vi "Main.vi"(0 "Start":bool, 1 "Temperature_Limit":T2={"Temperature_High_limit"=50.0, "Temperature_Low_Limit"=30.0} {"Temperature_Low_Limit" min=30.0 max=50.0 step=1.0; "Temperature_High_limit" min=30.0 max=50.0 step=1.0}, 2 "Current_Limit":T1={"Current_High_Limit"=120.0, "Current_Low_Limit"=100.0} {"Current_Low_Limit" min=100.0 max=120.0 step=1.0; "Current_High_Limit" min=100.0 max=120.0 step=1.0}, 5 "Stop":bool, 7 "Exit":bool, 9 "Log Rate":dbl, 11 "Error in":errorcluster) -> (4 "Temperature":i32, 6 "Current":i32, 8 "Waveform Graph":dbl[][](graph), 15 "Error out":errorcluster)   [LabVIEW 2020]
doc: "This system is used to get the current and temperature data which is generated and check if the generated data is in the specific range and generate error and the data is logged in the graph and the user can customize the the time on which the graph to be plotted"
uses:
  Controls/Temperature limit.ctl
  Controls/Current limit.ctl
  Typedefs/Data cluster.ctl
  Typedefs/Stop cases.ctl
panel:
  # "Data Acquisition and Monitoring"
  # "Press to start\nacquisition"
  # "Acquired data"
  # "Log rate \ncontrol"
  # "Press to stop\nacquisition"
  # "Press to \nterminate\nacquisition"
  # "Controls the\ndata limit"
  # "INPUT"
  # "OUTPUT"
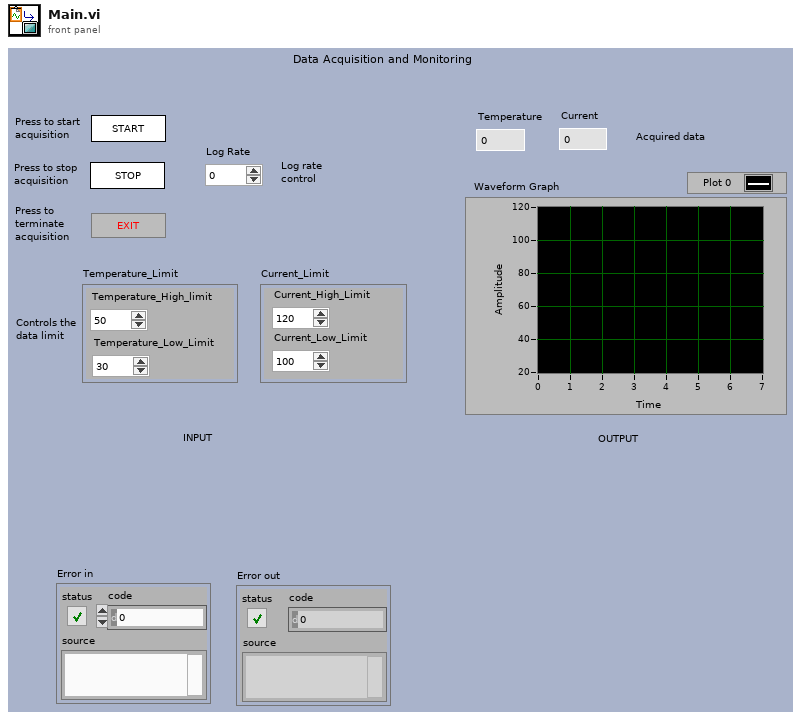
[diagram p1: front panel]
types:
  T1 = typedef "Current limit.ctl" = cluster{"Current_High_Limit":dbl, "Current_Low_Limit":dbl}
  T2 = typedef "Temperature limit.ctl" = cluster{"Temperature_High_limit":dbl, "Temperature_Low_Limit":dbl}
  T3 = typedef "Data cluster.ctl" = cluster{"Current":i32, "Temperature":i32}
  T4 = typedef "Stop cases.ctl" = enum16{"Initialize", "Write", "Stop"}
  T5 = enum8{"Enabled", "Disabled", "Disabled and Grayed Out"}
  T6 = enum32{"Bad", "Idle", "Run top level", "Running"}
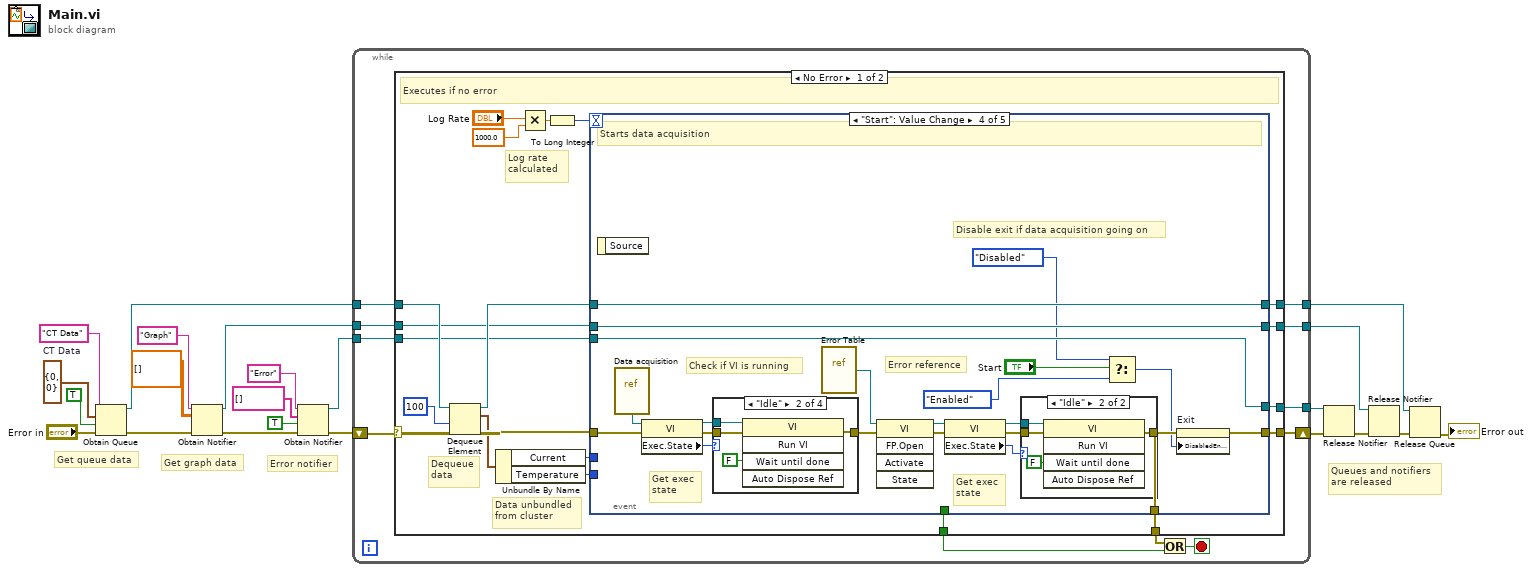
[diagram p0: block diagram]
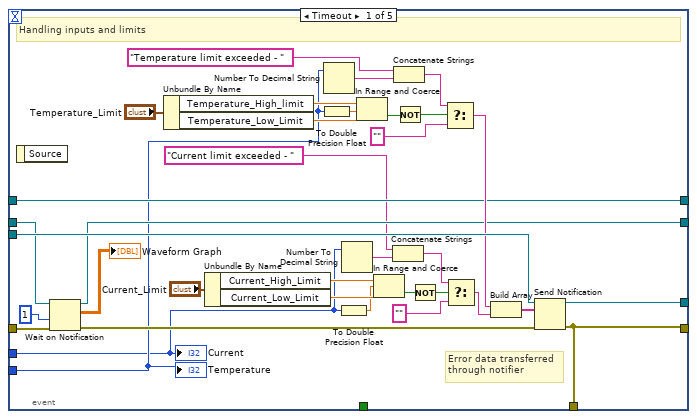
[diagram p2: hidden frame]
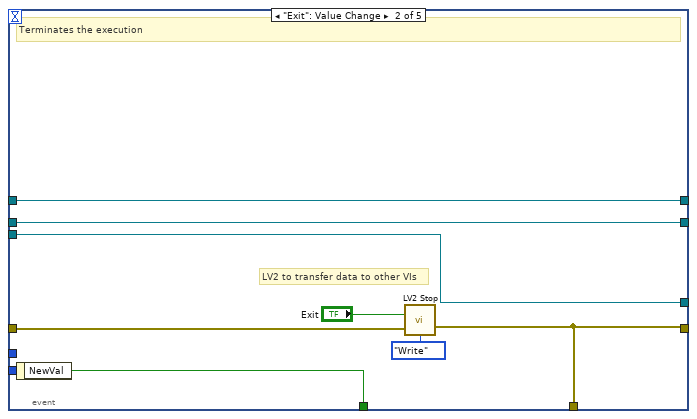
[diagram p3: hidden frame]
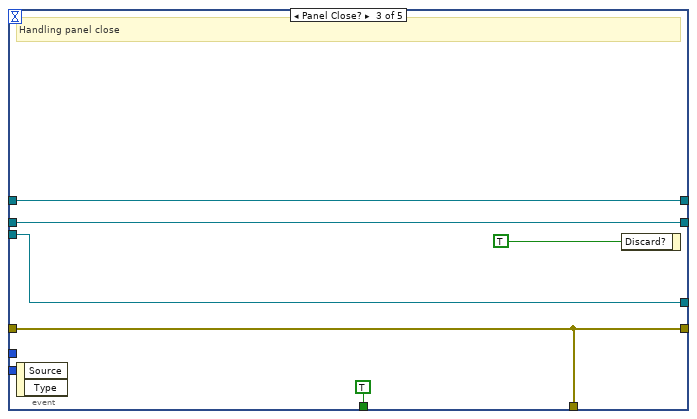
[diagram p4: hidden frame]
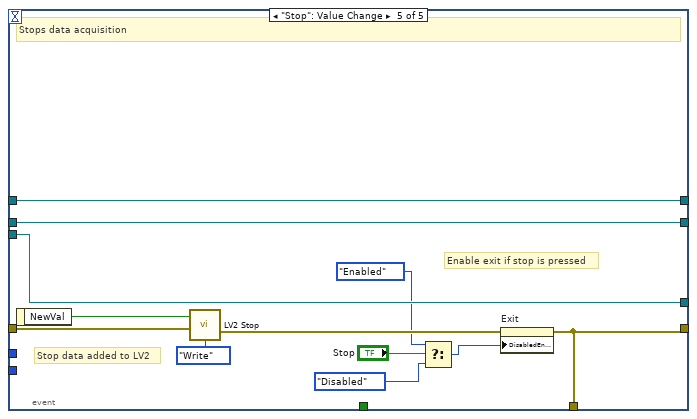
[diagram p9: hidden frame]
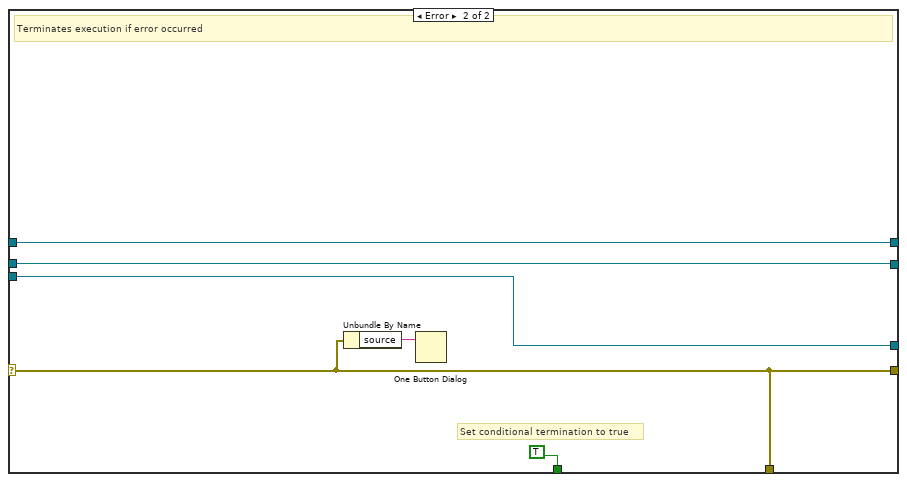
[diagram p10: hidden frame]
diagram:
  w20 = T3 {"Current"=0, "Temperature"=0}  # CT Data
  # "Error notifier"
  # "Get graph data"
  # "Queues and notifiers\nare released"
  # "Get queue data"
  n1 = Obtain Queue(name (unnamed)="CT Data", element data type=w20, create if not found? (T)=TRUE, error in (no error)="Error in") -> (queue out=w18:refnum<queue>, error out=w5:errorcluster)  [unwired: 1 in, 1 out]
  n2 = Obtain Notifier(name (unnamed)="Graph", notification data type=dbl[][] [], error in (no error)=w5) -> (notifier out=w2:refnum<notifier>, error out=w4:errorcluster)  [unwired: 1 in, 1 out]
  n3 = Obtain Notifier(name (unnamed)="Error", notification data type=string[] [], create if not found? (T)=TRUE, error in (no error)=w4) -> (notifier out=w1:refnum<notifier>, error out=w3:errorcluster)  [unwired: 1 out]
  n4 = while {
    shift-right: [w33] -> w17
    shift-left: w3 -> [w32]
    tunnel: [w27] -> w16
    tunnel: [w25] -> w11
    tunnel: w2 -> [w24]
    tunnel: w1 -> [w23]
    tunnel: w18 -> [w31]
    tunnel: [w26] -> w12
    stop <- w30 stop-if-true
    n5 = case shown="No Error" w32 {
      selector: w32 -> [w34 w152]
      tunnel: [w53 w152] -> w33
      tunnel: w31 -> [w49 w150]
      tunnel: [w52 TRUE ("NewVal")] -> w29
      tunnel: [w41 w152] -> w28
      tunnel: [w40 w148] -> w27
      tunnel: [w38 w150] -> w26
      tunnel: [w37 w149] -> w25
      tunnel: w24 -> [w36 w149]
      tunnel: w23 -> [w35 w148]
      frame No Error {
        # "Data unbundled\nfrom cluster"
        # "Dequeue\ndata"
        # "Log rate \ncalculated"
        # "Executes if no error"
        n6 = Dequeue Element(queue=w49, timeout in ms (-1)=100, error in (no error)=w34) -> (queue out=w39:refnum<queue>, element=w48:T3, error out=w50:errorcluster)  [unwired: 1 out]
        n7 = Unbundle By Name(w48) -> ("Current"=w47:i32, "Temperature"=w46:i32)
        n8 = Multiply(x="Log Rate", y=1000.0) -> (x*y=w44:dbl)
        n9 = To Long Integer(number=w44) -> (32bit integer=w45:i32)
        n10 = event shown="[3] \"Start\": Value Change" {
          selector: _ -> [_ _ _ _ _]
          dyn-events: _ -> [_ _ _ _ _]
          timeout: w45 -> [_ _ _ _ _]
          tunnel: w50 -> [w70 w89 w97 w122 w146]
          tunnel: [w62 w90 w97 w107 w140] -> w53
          tunnel: w35 -> [w84 w91 w100 w109 w142]
          tunnel: [_ w96 TRUE ("NewVal") _ _] -> w52
          tunnel: w47 -> [w55 _ _ _ _]
          tunnel: w46 -> [w61 _ _ _ _]
          tunnel: [w62 w90 w97 w108 w140] -> w41
          tunnel: w36 -> [w68 w92 w98 w110 w143]
          tunnel: [w66 w91 w100 w109 w142] -> w40
          tunnel: w39 -> [w64 w93 w99 w111 w144]
          tunnel: [w64 w93 w99 w111 w144] -> w38
          tunnel: [w65 w92 w98 w110 w143] -> w37
          event Timeout {
            # "Error data transferred \nthrough notifier"
            # "Handling inputs and limits"
            n11 = event-data() -> ()  [unwired: 1 in, 1 out]
            n12 = Wait on Notification(notifier=w68, timeout in ms (-1)=1, error in (no error)=w70) -> (notifier out=w65:refnum<notifier>, notification=→"Waveform Graph":dbl[][], error out=w69:errorcluster)  [unwired: 1 in, 1 out]
            n13 = Unbundle By Name("Temperature_Limit") -> ("Temperature_High_limit"=w80:dbl, "Temperature_Low_Limit"=w79:dbl)
            n14 = Unbundle By Name("Current_Limit") -> ("Current_High_Limit"=w77:dbl, "Current_Low_Limit"=w78:dbl)
            n15 = To Double Precision Float(number=w61) -> (double precision float=w71:dbl)
            n16 = Number To Decimal String(number=w61) -> (decimal integer string=w59:string)  [unwired: 1 in]
            n17 = To Double Precision Float(number=w55) -> (double precision float=w76:dbl)
            n18 = Number To Decimal String(number=w55) -> (decimal integer string=w57:string)  [unwired: 1 in]
            n19 = In Range and Coerce(upper limit=w80, x=w71, lower limit=w79) -> (In Range?=w75:bool)  [unwired: 1 out]
            n20 = In Range and Coerce(upper limit=w77, x=w76, lower limit=w78) -> (In Range?=w73:bool)  [unwired: 1 out]
            n21 = Concatenate Strings("Current limit exceeded - ", w57) -> (w54:string)
            n22 = Concatenate Strings("Temperature limit exceeded - ", w59) -> (w58:string)
            n23 = Not(x=w75) -> (.not. x?=w74:bool)
            n24 = Not(x=w73) -> (.not. x?=w72:bool)
            n25 = Select(t=w58, s=w74, f="") -> (s? t:f=w82:string)
            n26 = Select(t=w54, s=w72, f="") -> (s? t:f=w83:string)
            n27 = Build Array(w82, w83) -> (w81:string[])
            n28 = Send Notification(notification=w81, notifier=w84, error in (no error)=w69) -> (notifier out=w66:refnum<notifier>, error out=w62:errorcluster)
            "Temperature" <- w61
            "Current" <- w55
          }
          event "Exit": Value Change {
            # "LV2 to transfer data to other VIs"
            # "Terminates the execution"
            n29 = event-data() -> ("NewVal"=w96:bool)  [unwired: 1 in]
            n30 = call "LV2 Stop.vi"("Stop"="Exit", "Error in"=w89, "Operation"=Stop_cases."Write") -> ("Error out"=w90:errorcluster)  [unwired: 11 in, 1 out]
          }
          event Panel Close? {
            # "Handling panel close"
            n31 = event-data() -> ()  [unwired: 1 in, 2 out]
            n32 = event-data("Discard?"=TRUE) -> ()  [unwired: 1 in, 1 out]
          }
          event "Start": Value Change {
            # "Disable exit if data acquisition going on"
            # "Get exec \nstate"
            # "Error reference"
            # "Get exec \nstate"
            # "Check if VI is running"
            # "Starts data acquisition"
            n33 = event-data() -> ()  [unwired: 1 in, 1 out]
            n34 = vi-ref "Data acquisition.vi"() -> (w123:refnum<vi>)
            n35 = property class="VI"(reference=w123, error in=w122) -> (reference out=w119:refnum<vi>, error out=w121:errorcluster, "Exec.State"=w120:T6)
            n36 = case shown="\"Idle\"" w120 {
              tunnel: [w129 w131 w134 w135] -> w113
              tunnel: w121 -> [w129 w132 w134 w135]
              tunnel: w119 -> [_ w130 _ _]
              frame "Bad" {
              }
              frame "Idle" {
                n37 = invoke class="VI" method="Run VI"(reference=w130, error in=w132, "Wait until done"=FALSE ("Wait Until Done")) -> (error out=w131:errorcluster)  [unwired: 2 in, 4 out]
              }
              frame "Run top level" {
              }
              frame "Running" {
              }
            }
            n38 = vi-ref "Error Table.vi"() -> (w112:refnum<vi>)
            n39 = invoke class="VI" method="FP.Open"(reference=w112, error in=w113) -> (reference out=w115:refnum<vi>, error out=w114:errorcluster)  [unwired: 3 in, 3 out]
            n40 = property class="VI"(reference=w115, error in=w114) -> (reference out=w117:refnum<vi>, error out=w118:errorcluster, "Exec.State"=w116:T6)
            n41 = case shown="\"Idle\"" w116 {
              tunnel: [w124 w128] -> w108
              tunnel: w118 -> [w124 w127]
              tunnel: w117 -> [_ w126]
              frame "Bad", Default {
              }
              frame "Idle" {
                n42 = invoke class="VI" method="Run VI"(reference=w126, error in=w127, "Wait until done"=FALSE ("Wait Until Done")) -> (error out=w128:errorcluster)  [unwired: 2 in, 4 out]
              }
            }
            n43 = Select(t=T5."Disabled" ("Disabled"), s="Start", f=T5."Enabled" ("Disabled")) -> (s? t:f=w106:T5)
            n44 = property on="Exit" class="Bool"(error in=w108, "DisabledEnum"=w106) -> (error out=w107:errorcluster)  [unwired: 1 in, 1 out]
          }
          event "Stop": Value Change {
            # "Enable exit if stop is pressed"
            # "Stop data added to LV2"
            # "Stops data acquisition"
            n45 = event-data() -> ("NewVal"=w145:bool)  [unwired: 1 in]
            n46 = call "LV2 Stop.vi"("Stop"=w145, "Error in"=w146, "Operation"=Stop_cases."Write") -> ("Error out"=w141:errorcluster)  [unwired: 11 in, 1 out]
            n47 = Select(t=T5."Enabled" ("Disabled"), s="Stop", f=T5."Disabled" ("Disabled")) -> (s? t:f=w139:T5)
            n48 = property on="Exit" class="Bool"(error in=w141, "DisabledEnum"=w139) -> (error out=w140:errorcluster)  [unwired: 1 in, 1 out]
          }
        }
      }
      frame Error {
        # "Set conditional termination to true"
        # "Terminates execution if error occurred"
        n49 = Unbundle By Name(w152) -> ("source"=w153:string)
        n50 = One Button Dialog(message=w153) -> ()  [unwired: 1 in, 1 out]
      }
    }
    n51 = Or(x=w28, y=w29) -> (x .or. y?=w30:bool)
  }
  n52 = Release Notifier(notifier=w16, error in (no error)=w17) -> (error out=w15:errorcluster)  [unwired: 1 in, 2 out]
  n53 = Release Notifier(notifier=w11, error in (no error)=w15) -> (error out=w14:errorcluster)  [unwired: 1 in, 2 out]
  n54 = Release Queue(queue=w12, error in (no error)=w14) -> (error out=→"Error out":errorcluster)  [unwired: 1 in, 2 out]
